vi "Drive_Hardware_Begin.vi"() -> ()   [LabVIEW 2020]
uses:
  <vilib>/Rock Robotics/WPI/ThirdParty/Phoenix-LabVIEW/Motor Controller/Controls/CTRE_Phoenix_MotorControl_BaseConfigurables.ctl
  <vilib>/Rock Robotics/WPI/ThirdParty/Phoenix-LabVIEW/Motor Controller/Controls/CTRE_Phoenix_MotorControl_VelocityMeasurementPeriod.ctl
  <vilib>/Rock Robotics/WPI/ThirdParty/Phoenix-LabVIEW/Motor Controller/Controls/CTRE_Phoenix_MotorControl_SlotStructure.ctl
  <vilib>/Rock Robotics/WPI/ThirdParty/Phoenix-LabVIEW/Motor Controller/Controls/CTRE_Phoenix_MotorControl_FilterStruct.ctl
  <vilib>/Rock Robotics/WPI/ThirdParty/Phoenix-LabVIEW/Motor Controller/Controls/CTRE_Phoenix_MotorControl_RemoteSourceType.ctl
  <vilib>/Rock Robotics/WPI/ThirdParty/Phoenix-LabVIEW/Controls/CTRE_Phoenix_CustomParamConfiguration.ctl
  <vilib>/Rock Robotics/WPI/ThirdParty/Phoenix-LabVIEW/Motor Controller/Controls/CTRE_Phoenix_MotorControl_FeedbackDevice_TalonFX.ctl
  <vilib>/Rock Robotics/WPI/ThirdParty/Phoenix-LabVIEW/Motor Controller/Controls/CTRE_Phoenix_MotorControl_LimitSwitchNormal.ctl
  <vilib>/Rock Robotics/WPI/ThirdParty/Phoenix-LabVIEW/Motor Controller/Controls/CTRE_Phoenix_MotorControl_LimitSwitchSource_Local.ctl
  <vilib>/Rock Robotics/WPI/ThirdParty/Phoenix-LabVIEW/Motor Controller/Controls/CTRE_Phoenix_MotorControl_SupplyCurrentLimitConfiguration.ctl
  <vilib>/Rock Robotics/WPI/ThirdParty/Phoenix-LabVIEW/Motor Controller/Controls/CTRE_Phoenix_MotorControl_StatorCurrentLimitConfiguration.ctl
  <vilib>/Rock Robotics/WPI/ThirdParty/Phoenix-LabVIEW/Motor Controller/Controls/CTRE_Phoenix_MotorControl_MotorCommutation_TalonFX.ctl
  <vilib>/Rock Robotics/WPI/ThirdParty/Phoenix-LabVIEW/CANCoder/Controls/CTRE_Phoenix_CANcoder_AbsoluteSensorRange.ctl
  <vilib>/Rock Robotics/WPI/ThirdParty/Phoenix-LabVIEW/CANCoder/Controls/CTRE_Phoenix_CANcoder_SensorInitializationStrategy.ctl
  <vilib>/Rock Robotics/WPI/ThirdParty/Phoenix-LabVIEW/Motor Controller/Controls/CTRE_Phoenix_MotorControl_TalonFXInvertType.ctl
  <vilib>/Rock Robotics/WPI/ThirdParty/Phoenix-LabVIEW/Motor Controller/Controls/CTRE_Phoenix_MotorControl_NeutralMode.ctl
  <vilib>/Rock Robotics/WPI/ThirdParty/Phoenix-LabVIEW/Pigeon IMU/CTRE_PigeonIMU_Open_TalonSRX.vi
  Drive_Hardware_Globals.vi
panel:
  in  "Talon FX Configurables":T15={"Base Configurables"={"openLoopRamp"=0.0, "closedLoopRamp"=0.0, "peakOutputForward"=1.0, "peakOutputReverse"=-1.0, "nominalOutputForward"=0.0, "nominalOutputReverse"=0.0, "neutralDeadband"=0.0, "voltageCompSaturation"=0.0, "voltageMeasurementFilter"=32, "velocityMeasurementPeriod"=100, "velocityMeasurementWindow"=64, "forwardSoftLimitThreshold"=0, "reverseSoftLimitThreshold"=0, "forwardSoftLimitEnable"=FALSE, "reverseSoftLimitEnable"=FALSE, "slot0"={"P"=0.0, "I"=0.0, "D"=0.0, "F"=0.0, "integralZone"=0.0, "allowableClosedLoopError"=0, "maxIntegralAccumulator"=0.0, "closedLoopPeakOutput"=1.0, "closedLoopPeriod"=1}, "slot1"={"P"=0.0, "I"=0.0, "D"=0.0, "F"=0.0, "integralZone"=0.0, "allowableClosedLoopError"=0, "maxIntegralAccumulator"=0.0, "closedLoopPeakOutput"=1.0, "closedLoopPeriod"=1}, "slot2"={"P"=0.0, "I"=0.0, "D"=0.0, "F"=0.0, "integralZone"=0.0, "allowableClosedLoopError"=0, "maxIntegralAccumulator"=0.0, "closedLoopPeakOutput"=1.0, "closedLoopPeriod"=1}, "slot3"={"P"=0.0, "I"=0.0, "D"=0.0, "F"=0.0, "integralZone"=0.0, "allowableClosedLoopError"=0, "maxIntegralAccumulator"=0.0, "closedLoopPeakOutput"=1.0, "closedLoopPeriod"=1}, "auxPIDPolarity"=FALSE, "remoteFilter0"={"remoteSensorDeviceID"=0, "remoteSensorSource"=enum."Off"}, "remoteFilter1"={"remoteSensorDeviceID"=0, "remoteSensorSource"=enum."Off"}, "motionCruiseVelocity"=0, "motionAcceleration"=0, "motionProfileTrajectoryPeriod"=0, "feedbackNotContinuous"=FALSE, "remoteSensorClosedLoopDisableNeutralOnLOS"=FALSE, "clearPositionOnLimitF"=FALSE, "clearPositionOnLimitR"=FALSE, "clearPositionOnQuadIdx"=FALSE, "limitSwitchDisableNeutralOnLOS"=FALSE, "softLimitDisableNeutralOnLOS"=FALSE, "pulseWidthPeriod_EdgesPerRot"=1, "pulseWidthPeriod_FilterWindowSz"=1, "customParam"={"customParam0"=0, "customParam1"=0}, "trajectoryInterpolationEnable"=TRUE}, "primaryPID"={"selectedFeedbackCoefficient"=1.0, "selectedFeedbackSensor"=1}, "auxiliaryPID"={"selectedFeedbackCoefficient"=1.0, "selectedFeedbackSensor"=1}, "forwardLimitSwitchNormal"=enum."Normally Open", "reverseLimitSwitchNormal"=enum."Normally Open", "forwardLimitSwitchDeviceID"=0, "reverseLimitSwitchDeviceID"=0, "forwardLimitSwitchSource"=enum."Feedback Connector", "reverseLimitSwitchSource"=enum."Feedback Connector", "sum0Term"=1, "sum1Term"=1, "diff0Term"=1, "diff1Term"=1, "Supply Current Limit Configuration"={"Enable?"=FALSE, "Current Limit"=0.0, "Threshold Current"=0.0, "Threshold Time"=0.0}, "Stator Current Limit Configuration"={"Enable?"=FALSE, "Current Limit"=0.0, "Threshold Current"=0.0, "Threshold Time"=0.0}, "Motor Commutation"=enum."Trapezoidal", "Absolute Sensor Range"=enum."Unsigned [0 to 360)", "Integrated Sensor Offset (Degrees)"=0.0, "Sensor Initialization Strategy"=enum."Boot To Zero"} {"Base Configurables"."velocityMeasurementPeriod" items=["Period_1ms"=1, "Period_2ms"=2, "Period_5ms"=5, "Period_10ms"=10, "Period_20ms"=20, "Period_25ms"=25, "Period_50ms"=50, "Period_100ms"=100]; "primaryPID"."selectedFeedbackSensor" items=["Integrated Sensor"=1, "Sensor Sum (S0 + S1)"=9, "Sensor Difference (D0 - D1)"=10, "Remote Source 0"=11, "Remote Source 1"=12, "None"=14, "Software Emulated"=15]; "auxiliaryPID"."selectedFeedbackSensor" items=["Integrated Sensor"=1, "Sensor Sum (S0 + S1)"=9, "Sensor Difference (D0 - D1)"=10, "Remote Source 0"=11, "Remote Source 1"=12, "None"=14, "Software Emulated"=15]; "sum0Term" items=["Integrated Sensor"=1, "Sensor Sum (S0 + S1)"=9, "Sensor Difference (D0 - D1)"=10, "Remote Source 0"=11, "Remote Source 1"=12, "None"=14, "Software Emulated"=15]; "sum1Term" items=["Integrated Sensor"=1, "Sensor Sum (S0 + S1)"=9, "Sensor Difference (D0 - D1)"=10, "Remote Source 0"=11, "Remote Source 1"=12, "None"=14, "Software Emulated"=15]; "diff0Term" items=["Integrated Sensor"=1, "Sensor Sum (S0 + S1)"=9, "Sensor Difference (D0 - D1)"=10, "Remote Source 0"=11, "Remote Source 1"=12, "None"=14, "Software Emulated"=15]; "diff1Term" items=["Integrated Sensor"=1, "Sensor Sum (S0 + S1)"=9, "Sensor Difference (D0 - D1)"=10, "Remote Source 0"=11, "Remote Source 1"=12, "None"=14, "Software Emulated"=15]}
  # "False: Primary Output = PID[0] + PID[1]  ---  Auxiliary Output = PID[0] - PID[1]\nTrue:  Primary Output = PID[0] - PID[1] --- Auxiliary Output = PID[0] + PID[1]"
  # "Enable the motion profile executor to perform linear interpolation between profile points.  Defaults to True."
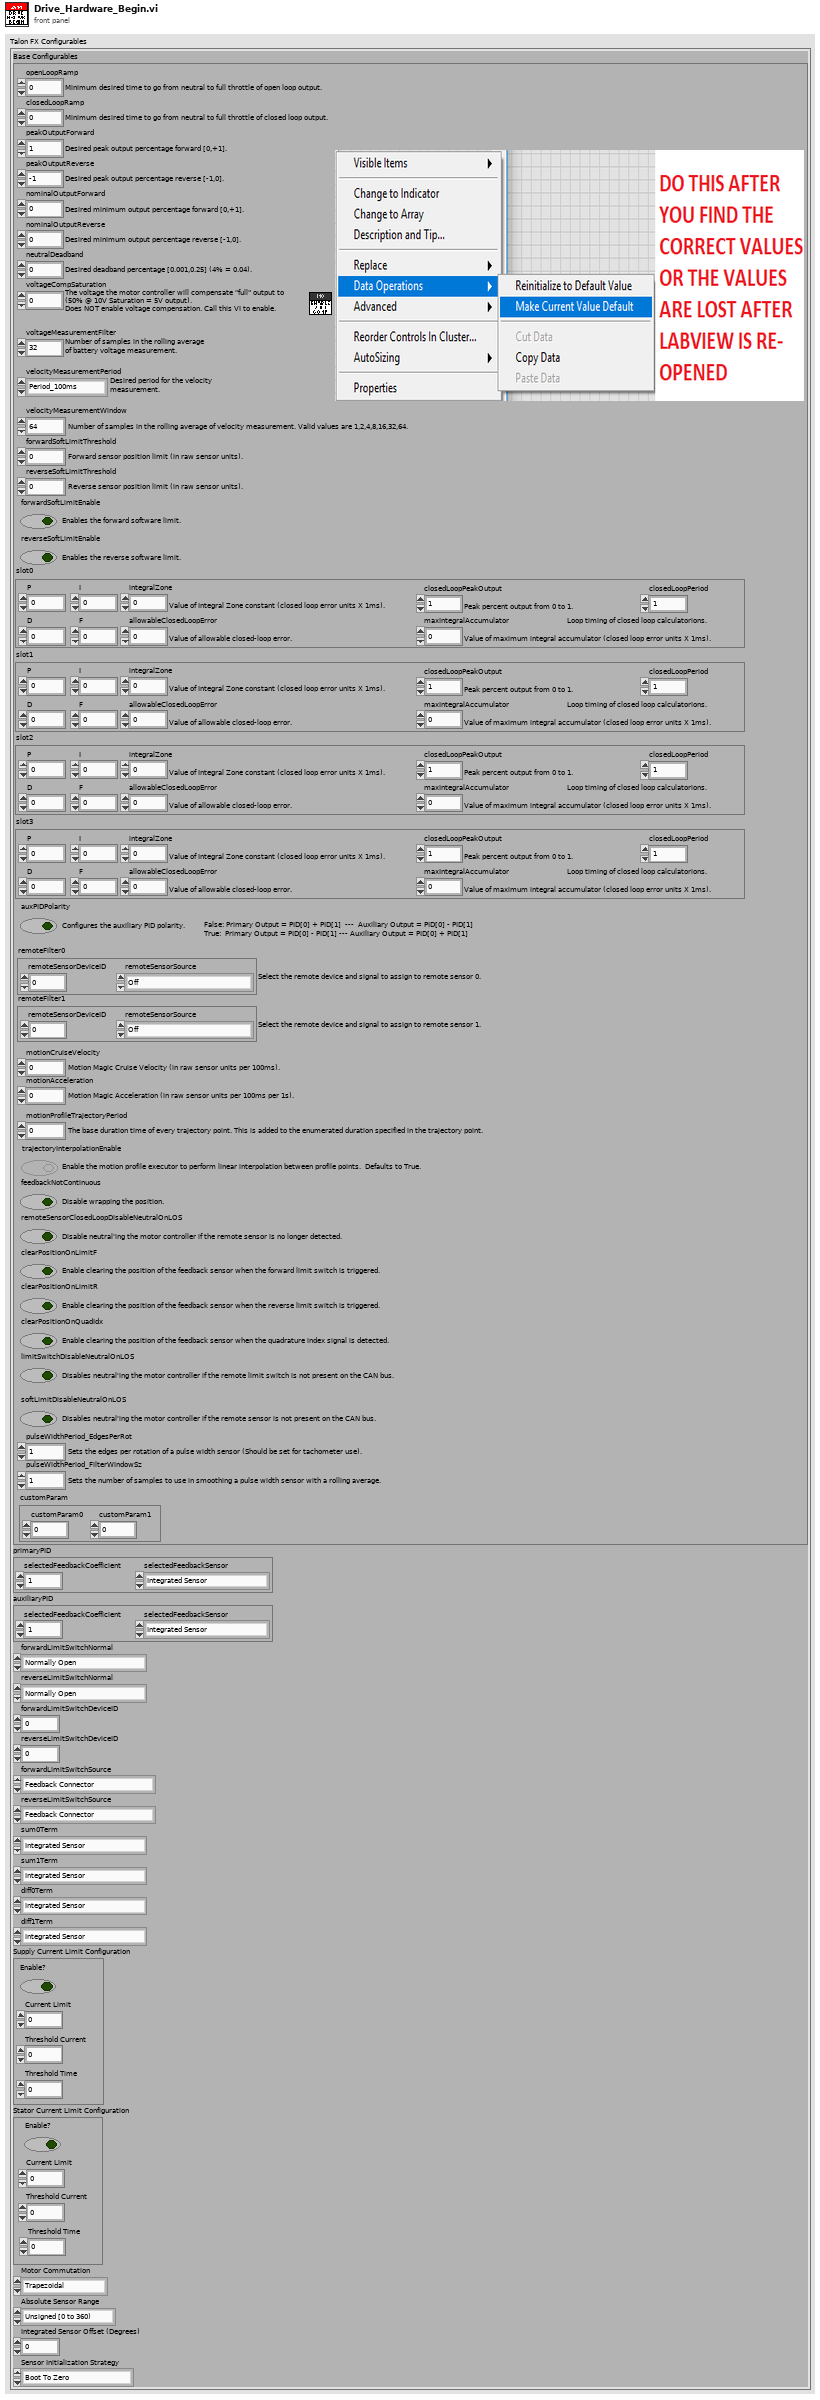
[diagram p1: front panel]
types:
  T1 = typedef "CTRE_Phoenix_MotorControl_BaseConfigurables.ctl" = cluster{"openLoopRamp":dbl, "closedLoopRamp":dbl, "peakOutputForward":dbl, "peakOutputReverse":dbl, "nominalOutputForward":dbl, "nominalOutputReverse":dbl, "neutralDeadband":dbl, "voltageCompSaturation":dbl, "voltageMeasurementFilter":i32, "velocityMeasurementPeriod":T2, "velocityMeasurementWindow":i32, "forwardSoftLimitThreshold":i32, "reverseSoftLimitThreshold":i32, "forwardSoftLimitEnable":bool, "reverseSoftLimitEnable":bool, "slot0":T3, "slot1":T3, "slot2":T3, "slot3":T3, "auxPIDPolarity":bool, "remoteFilter0":T4, "remoteFilter1":T4, "motionCruiseVelocity":i32, "motionAcceleration":i32, "motionProfileTrajectoryPeriod":i32, "feedbackNotContinuous":bool, "remoteSensorClosedLoopDisableNeutralOnLOS":bool, "clearPositionOnLimitF":bool, "clearPositionOnLimitR":bool, "clearPositionOnQuadIdx":bool, "limitSwitchDisableNeutralOnLOS":bool, "softLimitDisableNeutralOnLOS":bool, "pulseWidthPeriod_EdgesPerRot":i32, "pulseWidthPeriod_FilterWindowSz":i32, "customParam":T6, "trajectoryInterpolationEnable":bool}
  T2 = typedef "CTRE_Phoenix_MotorControl_VelocityMeasurementPeriod.ctl" = u16
  T3 = typedef "CTRE_Phoenix_MotorControl_SlotStructure.ctl" = cluster{"P":dbl, "I":dbl, "D":dbl, "F":dbl, "integralZone":dbl, "allowableClosedLoopError":i32, "maxIntegralAccumulator":dbl, "closedLoopPeakOutput":dbl, "closedLoopPeriod":i32}
  T4 = typedef "CTRE_Phoenix_MotorControl_FilterStruct.ctl" = cluster{"remoteSensorDeviceID":u8, "remoteSensorSource":T5}
  T5 = typedef "CTRE_Phoenix_MotorControl_RemoteSourceType.ctl" = enum16{"Off", "Talon SRX Selected Sensor", "Pigeon IMU Yaw", "Pigeon IMU Pitch", "Pigeon IMU Roll", "CANifier Quadrature", "CANifier PWM Input 0", "CANifier PWM Input 1", "CANifier PWM Input 2", "CANifier PWM Input 3", "Gadgeteer Pigeon Yaw", "Gadgeteer Pigeon Pitch", "Gadgeteer Pigeon Roll", "CANCoder"}
  T6 = typedef "CTRE_Phoenix_CustomParamConfiguration.ctl" = cluster{"customParam0":i32, "customParam1":i32}
  T7 = typedef "CTRE_Phoenix_MotorControl_FeedbackDevice_TalonFX.ctl" = i8
  T8 = typedef "CTRE_Phoenix_MotorControl_LimitSwitchNormal.ctl" = enum16{"Normally Open", "Normally Closed", "Disabled"}
  T9 = typedef "CTRE_Phoenix_MotorControl_LimitSwitchSource_Local.ctl" = enum16{"Feedback Connector", "Remote Talon SRX", "Remote CANifier", "Deactivated"}
  T10 = typedef "CTRE_Phoenix_MotorControl_SupplyCurrentLimitConfiguration.ctl" = cluster{"Enable?":bool, "Current Limit":dbl, "Threshold Current":dbl, "Threshold Time":dbl}
  T11 = typedef "CTRE_Phoenix_MotorControl_StatorCurrentLimitConfiguration.ctl" = cluster{"Enable?":bool, "Current Limit":dbl, "Threshold Current":dbl, "Threshold Time":dbl}
  T12 = typedef "CTRE_Phoenix_MotorControl_MotorCommutation_TalonFX.ctl" = enum16{"Trapezoidal"}
  T13 = typedef "CTRE_Phoenix_CANcoder_AbsoluteSensorRange.ctl" = enum16{"Unsigned [0 to 360)", "Signed [-180 to +180)"}
  T14 = typedef "CTRE_Phoenix_CANcoder_SensorInitializationStrategy.ctl" = enum16{"Boot To Zero", "Boot To Absolute Position"}
  T15 = cluster{"Base Configurables":T1, "primaryPID":cluster{"selectedFeedbackCoefficient":dbl, "selectedFeedbackSensor":T7}, "auxiliaryPID":cluster{"selectedFeedbackCoefficient":dbl, "selectedFeedbackSensor":T7}, "forwardLimitSwitchNormal":T8, "reverseLimitSwitchNormal":T8, "forwardLimitSwitchDeviceID":i32, "reverseLimitSwitchDeviceID":i32, "forwardLimitSwitchSource":T9, "reverseLimitSwitchSource":T9, "sum0Term":T7, "sum1Term":T7, "diff0Term":T7, "diff1Term":T7, "Supply Current Limit Configuration":T10, "Stator Current Limit Configuration":T11, "Motor Commutation":T12, "Absolute Sensor Range":T13, "Integrated Sensor Offset (Degrees)":dbl, "Sensor Initialization Strategy":T14}
  T16 = typedef "CTRE_Phoenix_MotorControl_TalonFXInvertType.ctl" = enum16{"Counter-Clockwise", "Clockwise"}
  T17 = typedef "CTRE_Phoenix_MotorControl_NeutralMode.ctl" = enum8{"EEPROMSetting", "Override to Coast", "Override to Brake"}
  T18 = typedef "WPI_MotorControlDeviceRef.ctl" = cluster{"DeviceStatus":errorcluster, "Type":T19, "PWM":cluster{"PWM Channel":T20, "DeadBand":T21}, "CAN":cluster{"Device Number":u8, "SetOutput VI Ref":variant, "GetOutput VI Ref":variant, "Enable VI Ref":variant, "Disable VI Ref":variant, "Data":variant}, "Invert":bool, "DIO PWM":cluster{"PWM \"Enable\" Channel":T20, "DIOChannel":T22, "PWM Rate":dbl}}
  T19 = typedef "WPI_MotorControlType.ctl" = enum16{"PWM", "CAN", "DIO PWM"}
  T20 = typedef "FPGA_DIOPWMChannel.ctl" = enum8{"PWM 0", "PWM 1", "PWM 2", "PWM 3", "PWM 4", "PWM 5", "PWM 6", "PWM 7", "PWM 8", "PWM 9", "PWM MXP 0", "PWM MXP 1", "PWM MXP 2", "PWM MXP 3", "PWM MXP 4", "PWM MXP 5", "PWM MXP 6", "PWM MXP 7", "PWM MXP 8", "PWM MXP 9", "Invalid"}
  T21 = typedef "WPI_PWMDeadband.ctl" = cluster{"Name":string, "maxPositivePwm":i32, "minPositivePwm":i32, "centerPwm":i32, "maxNegativePwm":i32, "minNegativePwm":i32, "angularRange":u16}
  T22 = typedef "FPGA_DIOChannel.ctl" = enum8{"DIO 0", "DIO 1", "DIO 2", "DIO 3", "DIO 4", "DIO 5", "DIO 6", "DIO 7", "DIO 8", "DIO 9", "DIO MXP 0", "DIO MXP 1", "DIO MXP 2", "DIO MXP 3", "DIO MXP 4", "DIO MXP 5", "DIO MXP 6", "DIO MXP 7", "DIO MXP 8", "DIO MXP 9", "DIO MXP 10", "DIO MXP 11", "DIO MXP 12", "DIO MXP 13", "DIO MXP 14", "DIO MXP 15", "SPI Port CS1", "SPI Port CS2", "SPI Port CS3", "SPI Port MISO", "SPI Port MOSI", "Invalid"}
  T23 = typedef "CTRE_PigeonIMU_DeviceRef.ctl" = cluster{"DeviceStatus":errorcluster, "Device Number":u8, "Type":T24, "Device ID":u32, "Handle":u64, "UsageFrame":u32, "Library Path":path}
  T24 = typedef "CTRE_PigeonIMU_ConnectionType.ctl" = u32
  T25 = typedef "CTRE_Phoenix_CANcoder_DeviceRef.ctl" = cluster{"DeviceStatus":errorcluster, "Device Number":u8, "Handle":u64, "UsageFrame":u32, "Library Path":path}
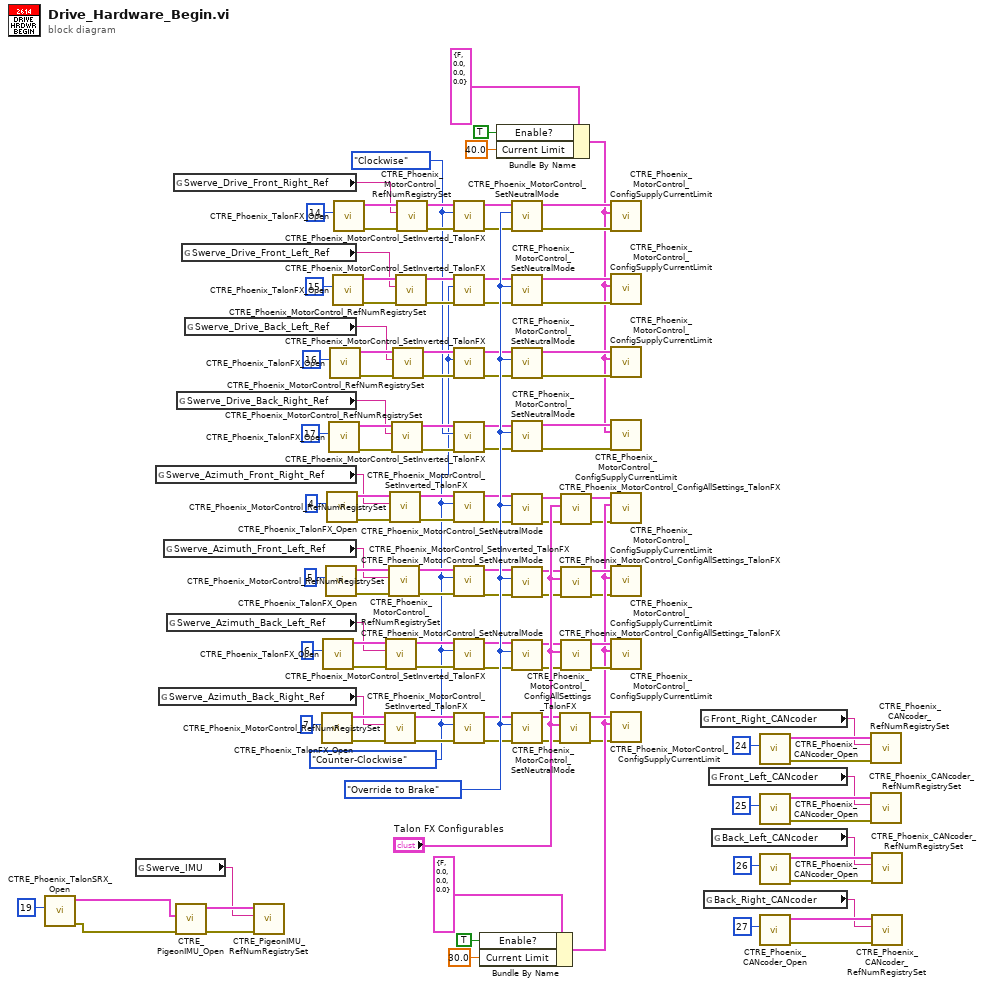
[diagram p0: block diagram]
diagram:
  w18 = CTRE_Phoenix_MotorControl_TalonFXInvertType."Clockwise" ("Invert Type")
  w110 = CTRE_Phoenix_MotorControl_NeutralMode."Override to Brake" ("Motor Control Neutral Mode")
  w17 = CTRE_Phoenix_MotorControl_TalonFXInvertType."Counter-Clockwise" ("Invert Type")
  n1 = call <vilib>:"CTRE_Phoenix_TalonSRX_Open.vi"("Device Number"=u8 19) -> ("error out"=w113:errorcluster, "PhoenixMotorControlDevRef"=w112:T18)  [unwired: 9 in]
  n2 = global read "Drive_Hardware_Globals.vi" "Swerve_IMU"() -> (w51:string)
  n3 = global read "Drive_Hardware_Globals.vi" "Swerve_Azimuth_Front_Right_Ref"() -> (w46:string)
  n4 = global read "Drive_Hardware_Globals.vi" "Swerve_Azimuth_Back_Right_Ref"() -> (w43:string)
  n5 = global read "Drive_Hardware_Globals.vi" "Swerve_Azimuth_Front_Left_Ref"() -> (w45:string)
  n6 = global read "Drive_Hardware_Globals.vi" "Swerve_Azimuth_Back_Left_Ref"() -> (w44:string)
  n7 = global read "Drive_Hardware_Globals.vi" "Swerve_Drive_Front_Right_Ref"() -> (w50:string)
  n8 = call-poly <vilib>:"CTRE_PigeonIMU_Open.vi"("error in"=w113, "CAN Talon SRX Ref"=w112) -> ("error out"=w53:errorcluster, "PigeonIMUDevRef"=w52:T23)  [unwired: 8 in]
  n9 = global read "Drive_Hardware_Globals.vi" "Swerve_Drive_Back_Right_Ref"() -> (w47:string)
  n10 = global read "Drive_Hardware_Globals.vi" "Swerve_Drive_Front_Left_Ref"() -> (w49:string)
  n11 = global read "Drive_Hardware_Globals.vi" "Swerve_Drive_Back_Left_Ref"() -> (w48:string)
  n12 = call <vilib>:"CTRE_PigeonIMU_RefNumRegistrySet.vi"("error in (no error)"=w53, "refnum name"=w51, "PigeonIMUDevRef"=w52) -> ()  [unwired: 7 in, 2 out]
  n13 = call <vilib>:"CTRE_Phoenix_TalonFX_Open.vi"("Device Number"=u8 7) -> ("error out"=w80:errorcluster, "PhoenixMotorControlDevRef"=w83:T18)  [unwired: 9 in]
  n14 = call <vilib>:"CTRE_Phoenix_TalonFX_Open.vi"("Device Number"=u8 6) -> ("error out"=w77:errorcluster, "PhoenixMotorControlDevRef"=w74:T18)  [unwired: 9 in]
  n15 = call <vilib>:"CTRE_Phoenix_TalonFX_Open.vi"("Device Number"=u8 5) -> ("error out"=w87:errorcluster, "PhoenixMotorControlDevRef"=w84:T18)  [unwired: 9 in]
  n16 = call <vilib>:"CTRE_Phoenix_TalonFX_Open.vi"("Device Number"=u8 4) -> ("error out"=w90:errorcluster, "PhoenixMotorControlDevRef"=w93:T18)  [unwired: 9 in]
  n17 = call <vilib>:"CTRE_Phoenix_TalonFX_Open.vi"("Device Number"=u8 17) -> ("error out"=w67:errorcluster, "PhoenixMotorControlDevRef"=w64:T18)  [unwired: 9 in]
  n18 = call <vilib>:"CTRE_Phoenix_TalonFX_Open.vi"("Device Number"=u8 16) -> ("error out"=w70:errorcluster, "PhoenixMotorControlDevRef"=w73:T18)  [unwired: 9 in]
  n19 = call <vilib>:"CTRE_Phoenix_TalonFX_Open.vi"("Device Number"=u8 15) -> ("error out"=w60:errorcluster, "PhoenixMotorControlDevRef"=w63:T18)  [unwired: 9 in]
  n20 = call <vilib>:"CTRE_Phoenix_TalonFX_Open.vi"("Device Number"=u8 14) -> ("error out"=w57:errorcluster, "PhoenixMotorControlDevRef"=w54:T18)  [unwired: 9 in]
  n21 = call <vilib>:"CTRE_Phoenix_MotorControl_RefNumRegistrySet.vi"("error in (no error)"=w80, "refnum name"=w43, "PhoenixMotorControlDevRef"=w83) -> ("error out"=w81:errorcluster, "PhoenixMotorControlDevRef"=w82:T18)  [unwired: 7 in]
  n22 = call <vilib>:"CTRE_Phoenix_MotorControl_RefNumRegistrySet.vi"("error in (no error)"=w77, "refnum name"=w44, "PhoenixMotorControlDevRef"=w74) -> ("error out"=w76:errorcluster, "PhoenixMotorControlDevRef"=w75:T18)  [unwired: 7 in]
  n23 = call <vilib>:"CTRE_Phoenix_MotorControl_RefNumRegistrySet.vi"("error in (no error)"=w87, "refnum name"=w45, "PhoenixMotorControlDevRef"=w84) -> ("error out"=w86:errorcluster, "PhoenixMotorControlDevRef"=w85:T18)  [unwired: 7 in]
  n24 = call <vilib>:"CTRE_Phoenix_MotorControl_RefNumRegistrySet.vi"("error in (no error)"=w90, "refnum name"=w46, "PhoenixMotorControlDevRef"=w93) -> ("error out"=w91:errorcluster, "PhoenixMotorControlDevRef"=w92:T18)  [unwired: 7 in]
  n25 = call <vilib>:"CTRE_Phoenix_MotorControl_RefNumRegistrySet.vi"("error in (no error)"=w67, "refnum name"=w47, "PhoenixMotorControlDevRef"=w64) -> ("error out"=w66:errorcluster, "PhoenixMotorControlDevRef"=w65:T18)  [unwired: 7 in]
  n26 = call <vilib>:"CTRE_Phoenix_MotorControl_RefNumRegistrySet.vi"("error in (no error)"=w70, "refnum name"=w48, "PhoenixMotorControlDevRef"=w73) -> ("error out"=w71:errorcluster, "PhoenixMotorControlDevRef"=w72:T18)  [unwired: 7 in]
  n27 = call <vilib>:"CTRE_Phoenix_MotorControl_RefNumRegistrySet.vi"("error in (no error)"=w60, "refnum name"=w49, "PhoenixMotorControlDevRef"=w63) -> ("error out"=w61:errorcluster, "PhoenixMotorControlDevRef"=w62:T18)  [unwired: 7 in]
  n28 = call <vilib>:"CTRE_Phoenix_MotorControl_RefNumRegistrySet.vi"("error in (no error)"=w57, "refnum name"=w50, "PhoenixMotorControlDevRef"=w54) -> ("error out"=w56:errorcluster, "PhoenixMotorControlDevRef"=w55:T18)  [unwired: 7 in]
  n29 = call <vilib>:"CTRE_Phoenix_MotorControl_SetInverted_TalonFX.vi"("error in (no error)"=w56, "Invert Type"=w18, "PhoenixMotorControlDevRef"=w55) -> ("error out"=w97:errorcluster, "PhoenixMotorControlDevRef"=w96:T18)  [unwired: 7 in]
  n30 = call <vilib>:"CTRE_Phoenix_MotorControl_SetInverted_TalonFX.vi"("error in (no error)"=w61, "Invert Type"=w17, "PhoenixMotorControlDevRef"=w62) -> ("error out"=w99:errorcluster, "PhoenixMotorControlDevRef"=w98:T18)  [unwired: 7 in]
  n31 = call <vilib>:"CTRE_Phoenix_MotorControl_SetInverted_TalonFX.vi"("error in (no error)"=w71, "Invert Type"=w17, "PhoenixMotorControlDevRef"=w72) -> ("error out"=w101:errorcluster, "PhoenixMotorControlDevRef"=w100:T18)  [unwired: 7 in]
  n32 = call <vilib>:"CTRE_Phoenix_MotorControl_SetInverted_TalonFX.vi"("error in (no error)"=w66, "Invert Type"=w18, "PhoenixMotorControlDevRef"=w65) -> ("error out"=w103:errorcluster, "PhoenixMotorControlDevRef"=w102:T18)  [unwired: 7 in]
  n33 = call <vilib>:"CTRE_Phoenix_MotorControl_SetInverted_TalonFX.vi"("error in (no error)"=w91, "Invert Type"=w17, "PhoenixMotorControlDevRef"=w92) -> ("error out"=w105:errorcluster, "PhoenixMotorControlDevRef"=w104:T18)  [unwired: 7 in]
  n34 = call <vilib>:"CTRE_Phoenix_MotorControl_SetInverted_TalonFX.vi"("error in (no error)"=w86, "Invert Type"=w17, "PhoenixMotorControlDevRef"=w85) -> ("error out"=w107:errorcluster, "PhoenixMotorControlDevRef"=w106:T18)  [unwired: 7 in]
  n35 = call <vilib>:"CTRE_Phoenix_MotorControl_SetInverted_TalonFX.vi"("error in (no error)"=w76, "Invert Type"=w17, "PhoenixMotorControlDevRef"=w75) -> ("error out"=w109:errorcluster, "PhoenixMotorControlDevRef"=w108:T18)  [unwired: 7 in]
  n36 = call <vilib>:"CTRE_Phoenix_MotorControl_SetInverted_TalonFX.vi"("error in (no error)"=w81, "Invert Type"=w17, "PhoenixMotorControlDevRef"=w82) -> ("error out"=w95:errorcluster, "PhoenixMotorControlDevRef"=w94:T18)  [unwired: 7 in]
  n37 = Bundle By Name(cluster=T10 {"Enable?"=FALSE, "Current Limit"=0.0, "Threshold Current"=0.0, "Threshold Time"=0.0} ("Supply Current Limit Configuration"), "Enable?"=TRUE, "Current Limit"=30.0) -> (w30:T10)
  n38 = Bundle By Name(cluster=T10 {"Enable?"=FALSE, "Current Limit"=0.0, "Threshold Current"=0.0, "Threshold Time"=0.0} ("Supply Current Limit Configuration"), "Enable?"=TRUE, "Current Limit"=40.0) -> (w19:T10)
  n39 = call <vilib>:"CTRE_Phoenix_MotorControl_SetNeutralMode.vi"("error in (no error)"=w97, "Motor Control Neutral Mode"=w110, "PhoenixMotorControlDevRef"=w96) -> ("error out"=w26:errorcluster, "PhoenixMotorControlDevRef"=w40:T18)  [unwired: 7 in]
  n40 = call <vilib>:"CTRE_Phoenix_MotorControl_SetNeutralMode.vi"("error in (no error)"=w99, "Motor Control Neutral Mode"=w110, "PhoenixMotorControlDevRef"=w98) -> ("error out"=w27:errorcluster, "PhoenixMotorControlDevRef"=w39:T18)  [unwired: 7 in]
  n41 = call <vilib>:"CTRE_Phoenix_MotorControl_SetNeutralMode.vi"("error in (no error)"=w101, "Motor Control Neutral Mode"=w110, "PhoenixMotorControlDevRef"=w100) -> ("error out"=w28:errorcluster, "PhoenixMotorControlDevRef"=w38:T18)  [unwired: 7 in]
  n42 = call <vilib>:"CTRE_Phoenix_MotorControl_SetNeutralMode.vi"("error in (no error)"=w103, "Motor Control Neutral Mode"=w110, "PhoenixMotorControlDevRef"=w102) -> ("error out"=w29:errorcluster, "PhoenixMotorControlDevRef"=w37:T18)  [unwired: 7 in]
  n43 = call <vilib>:"CTRE_Phoenix_MotorControl_SetNeutralMode.vi"("error in (no error)"=w105, "Motor Control Neutral Mode"=w110, "PhoenixMotorControlDevRef"=w104) -> ("error out"=w120:errorcluster, "PhoenixMotorControlDevRef"=w121:T18)  [unwired: 7 in]
  n44 = call <vilib>:"CTRE_Phoenix_MotorControl_SetNeutralMode.vi"("error in (no error)"=w107, "Motor Control Neutral Mode"=w110, "PhoenixMotorControlDevRef"=w106) -> ("error out"=w118:errorcluster, "PhoenixMotorControlDevRef"=w119:T18)  [unwired: 7 in]
  n45 = call <vilib>:"CTRE_Phoenix_MotorControl_SetNeutralMode.vi"("error in (no error)"=w109, "Motor Control Neutral Mode"=w110, "PhoenixMotorControlDevRef"=w108) -> ("error out"=w117:errorcluster, "PhoenixMotorControlDevRef"=w116:T18)  [unwired: 7 in]
  n46 = call <vilib>:"CTRE_Phoenix_MotorControl_SetNeutralMode.vi"("error in (no error)"=w95, "Motor Control Neutral Mode"=w110, "PhoenixMotorControlDevRef"=w94) -> ("error out"=w115:errorcluster, "PhoenixMotorControlDevRef"=w114:T18)  [unwired: 7 in]
  n47 = call <vilib>:"CTRE_Phoenix_MotorControl_ConfigAllSettings_TalonFX.vi"("error in (no error)"=w115, "Talon FX Configurables"="Talon FX Configurables", "PhoenixMotorControlDevRef"=w114) -> ("error out"=w23:errorcluster, "PhoenixMotorControlDevRef"=w34:T18)  [unwired: 7 in]
  n48 = call <vilib>:"CTRE_Phoenix_MotorControl_ConfigAllSettings_TalonFX.vi"("error in (no error)"=w120, "Talon FX Configurables"="Talon FX Configurables", "PhoenixMotorControlDevRef"=w121) -> ("error out"=w25:errorcluster, "PhoenixMotorControlDevRef"=w36:T18)  [unwired: 7 in]
  n49 = call <vilib>:"CTRE_Phoenix_MotorControl_ConfigAllSettings_TalonFX.vi"("error in (no error)"=w118, "Talon FX Configurables"="Talon FX Configurables", "PhoenixMotorControlDevRef"=w119) -> ("error out"=w24:errorcluster, "PhoenixMotorControlDevRef"=w35:T18)  [unwired: 7 in]
  n50 = call <vilib>:"CTRE_Phoenix_MotorControl_ConfigAllSettings_TalonFX.vi"("error in (no error)"=w117, "Talon FX Configurables"="Talon FX Configurables", "PhoenixMotorControlDevRef"=w116) -> ("error out"=w42:errorcluster, "PhoenixMotorControlDevRef"=w41:T18)  [unwired: 7 in]
  n51 = call <vilib>:"CTRE_Phoenix_MotorControl_ConfigSupplyCurrentLimit.vi"("error in (no error)"=w26, "Supply Current Limit Configuration"=w19, "PhoenixMotorControlDevRef"=w40) -> ()  [unwired: 7 in, 2 out]
  n52 = call <vilib>:"CTRE_Phoenix_MotorControl_ConfigSupplyCurrentLimit.vi"("error in (no error)"=w27, "Supply Current Limit Configuration"=w19, "PhoenixMotorControlDevRef"=w39) -> ()  [unwired: 7 in, 2 out]
  n53 = call <vilib>:"CTRE_Phoenix_MotorControl_ConfigSupplyCurrentLimit.vi"("error in (no error)"=w28, "Supply Current Limit Configuration"=w19, "PhoenixMotorControlDevRef"=w38) -> ()  [unwired: 7 in, 2 out]
  n54 = call <vilib>:"CTRE_Phoenix_MotorControl_ConfigSupplyCurrentLimit.vi"("error in (no error)"=w29, "Supply Current Limit Configuration"=w19, "PhoenixMotorControlDevRef"=w37) -> ()  [unwired: 7 in, 2 out]
  n55 = call <vilib>:"CTRE_Phoenix_MotorControl_ConfigSupplyCurrentLimit.vi"("error in (no error)"=w25, "Supply Current Limit Configuration"=w30, "PhoenixMotorControlDevRef"=w36) -> ()  [unwired: 7 in, 2 out]
  n56 = call <vilib>:"CTRE_Phoenix_MotorControl_ConfigSupplyCurrentLimit.vi"("error in (no error)"=w24, "Supply Current Limit Configuration"=w30, "PhoenixMotorControlDevRef"=w35) -> ()  [unwired: 7 in, 2 out]
  n57 = call <vilib>:"CTRE_Phoenix_MotorControl_ConfigSupplyCurrentLimit.vi"("error in (no error)"=w42, "Supply Current Limit Configuration"=w30, "PhoenixMotorControlDevRef"=w41) -> ()  [unwired: 7 in, 2 out]
  n58 = call <vilib>:"CTRE_Phoenix_MotorControl_ConfigSupplyCurrentLimit.vi"("error in (no error)"=w23, "Supply Current Limit Configuration"=w30, "PhoenixMotorControlDevRef"=w34) -> ()  [unwired: 7 in, 2 out]
  n59 = global read "Drive_Hardware_Globals.vi" "Front_Right_CANcoder"() -> (w4:string)
  n60 = global read "Drive_Hardware_Globals.vi" "Back_Right_CANcoder"() -> (w1:string)
  n61 = global read "Drive_Hardware_Globals.vi" "Front_Left_CANcoder"() -> (w3:string)
  n62 = global read "Drive_Hardware_Globals.vi" "Back_Left_CANcoder"() -> (w2:string)
  n63 = call <vilib>:"CTRE_Phoenix_CANcoder_Open.vi"("Device Number"=u8 24) -> ("error out"=w11:errorcluster, "CTRE_CANcoder_DeviceRef"=w12:T25)  [unwired: 9 in]
  n64 = call <vilib>:"CTRE_Phoenix_CANcoder_Open.vi"("Device Number"=u8 25) -> ("error out"=w9:errorcluster, "CTRE_CANcoder_DeviceRef"=w10:T25)  [unwired: 9 in]
  n65 = call <vilib>:"CTRE_Phoenix_CANcoder_Open.vi"("Device Number"=u8 26) -> ("error out"=w7:errorcluster, "CTRE_CANcoder_DeviceRef"=w8:T25)  [unwired: 9 in]
  n66 = call <vilib>:"CTRE_Phoenix_CANcoder_Open.vi"("Device Number"=u8 27) -> ("error out"=w5:errorcluster, "CTRE_CANcoder_DeviceRef"=w6:T25)  [unwired: 9 in]
  n67 = call <vilib>:"CTRE_Phoenix_CANcoder_RefNumRegistrySet.vi"("error in (no error)"=w11, "refnum name"=w4, "CTRE_CANcoder_DeviceRef"=w12) -> ()  [unwired: 7 in, 2 out]
  n68 = call <vilib>:"CTRE_Phoenix_CANcoder_RefNumRegistrySet.vi"("error in (no error)"=w9, "refnum name"=w3, "CTRE_CANcoder_DeviceRef"=w10) -> ()  [unwired: 7 in, 2 out]
  n69 = call <vilib>:"CTRE_Phoenix_CANcoder_RefNumRegistrySet.vi"("error in (no error)"=w7, "refnum name"=w2, "CTRE_CANcoder_DeviceRef"=w8) -> ()  [unwired: 7 in, 2 out]
  n70 = call <vilib>:"CTRE_Phoenix_CANcoder_RefNumRegistrySet.vi"("error in (no error)"=w5, "refnum name"=w1, "CTRE_CANcoder_DeviceRef"=w6) -> ()  [unwired: 7 in, 2 out]
